vi "5492_AutonomousTurnButBetter.vi"(8 "error in (no error)":errorcluster, 10 "Yaw Goallll":dbl) -> (0 "error out (no error)":errorcluster)   [LabVIEW 2017]
uses:
  <vilib>/Rock Robotics/WPI/ThirdParty/Cross The Road Electronics/Phoenix-LabVIEW/Motor Controller/Controls/CTRE_Phoenix_MotorControl_ControlMode.ctl
  <vilib>/Rock Robotics/WPI/Utilities/WPI_GetSetVariantRefNum.vi
  5492_InitialYaw.vi
  <vilib>/Rock Robotics/WPI/RobotDrive/WPI_RobotDriveSafetyCheck.vi
  5492_DriveRamp.vi
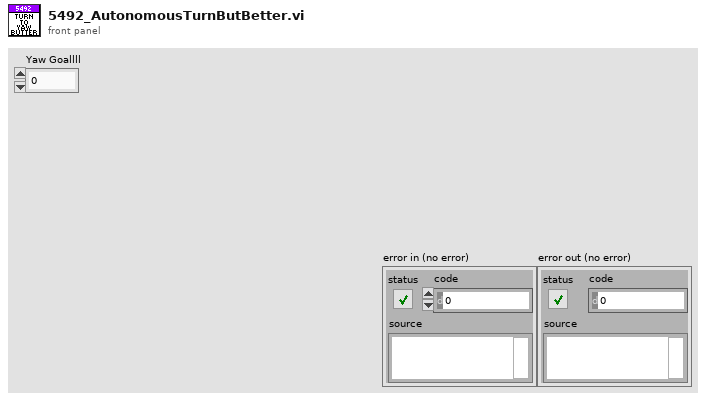
[diagram p1: front panel]
types:
  T1 = typedef "CTRE_Phoenix_MotorControl_ControlMode.ctl" = u16
  T2 = cluster{"Yaw":dbl, "Roll":dbl, "Pitch":dbl, "Heading":dbl, "Fused Heading":dbl}
  T3 = typedef "WPI_RobotDriveDevRef.ctl" = cluster{"DevStatus":errorcluster, "Motors[]":T4[], "Square Inputs":bool, "Max Output":dbl}
  T4 = typedef "WPI_MotorControlDeviceRef.ctl" = cluster{"DeviceStatus":errorcluster, "Type":T5, "PWM":cluster{"PWM Channel":T6, "DeadBand":T7}, "CAN":cluster{"Device Number":u8, "SetOutput VI Ref":variant, "GetOutput VI Ref":variant, "Enable VI Ref":variant, "Disable VI Ref":variant, "Data":variant}, "Invert":bool, "DIO PWM":cluster{"PWM \"Enable\" Channel":T6, "DIOChannel":T8, "PWM Rate":dbl}}
  T5 = typedef "WPI_MotorControlType.ctl" = enum16{"PWM", "CAN", "DIO PWM"}
  T6 = typedef "FPGA_DIOPWMChannel.ctl" = enum8{"PWM 0", "PWM 1", "PWM 2", "PWM 3", "PWM 4", "PWM 5", "PWM 6", "PWM 7", "PWM 8", "PWM 9", "PWM MXP 0", "PWM MXP 1", "PWM MXP 2", "PWM MXP 3", "PWM MXP 4", "PWM MXP 5", "PWM MXP 6", "PWM MXP 7", "PWM MXP 8", "PWM MXP 9", "Invalid"}
  T7 = typedef "WPI_PWMDeadband.ctl" = cluster{"Name":string, "maxPositivePwm":i32, "minPositivePwm":i32, "centerPwm":i32, "maxNegativePwm":i32, "minNegativePwm":i32, "angularRange":u16}
  T8 = typedef "FPGA_DIOChannel.ctl" = enum8{"DIO 0", "DIO 1", "DIO 2", "DIO 3", "DIO 4", "DIO 5", "DIO 6", "DIO 7", "DIO 8", "DIO 9", "DIO MXP 0", "DIO MXP 1", "DIO MXP 2", "DIO MXP 3", "DIO MXP 4", "DIO MXP 5", "DIO MXP 6", "DIO MXP 7", "DIO MXP 8", "DIO MXP 9", "DIO MXP 10", "DIO MXP 11", "DIO MXP 12", "DIO MXP 13", "DIO MXP 14", "DIO MXP 15", "SPI Port CS1", "SPI Port CS2", "SPI Port CS3", "SPI Port MISO", "SPI Port MOSI", "Invalid"}
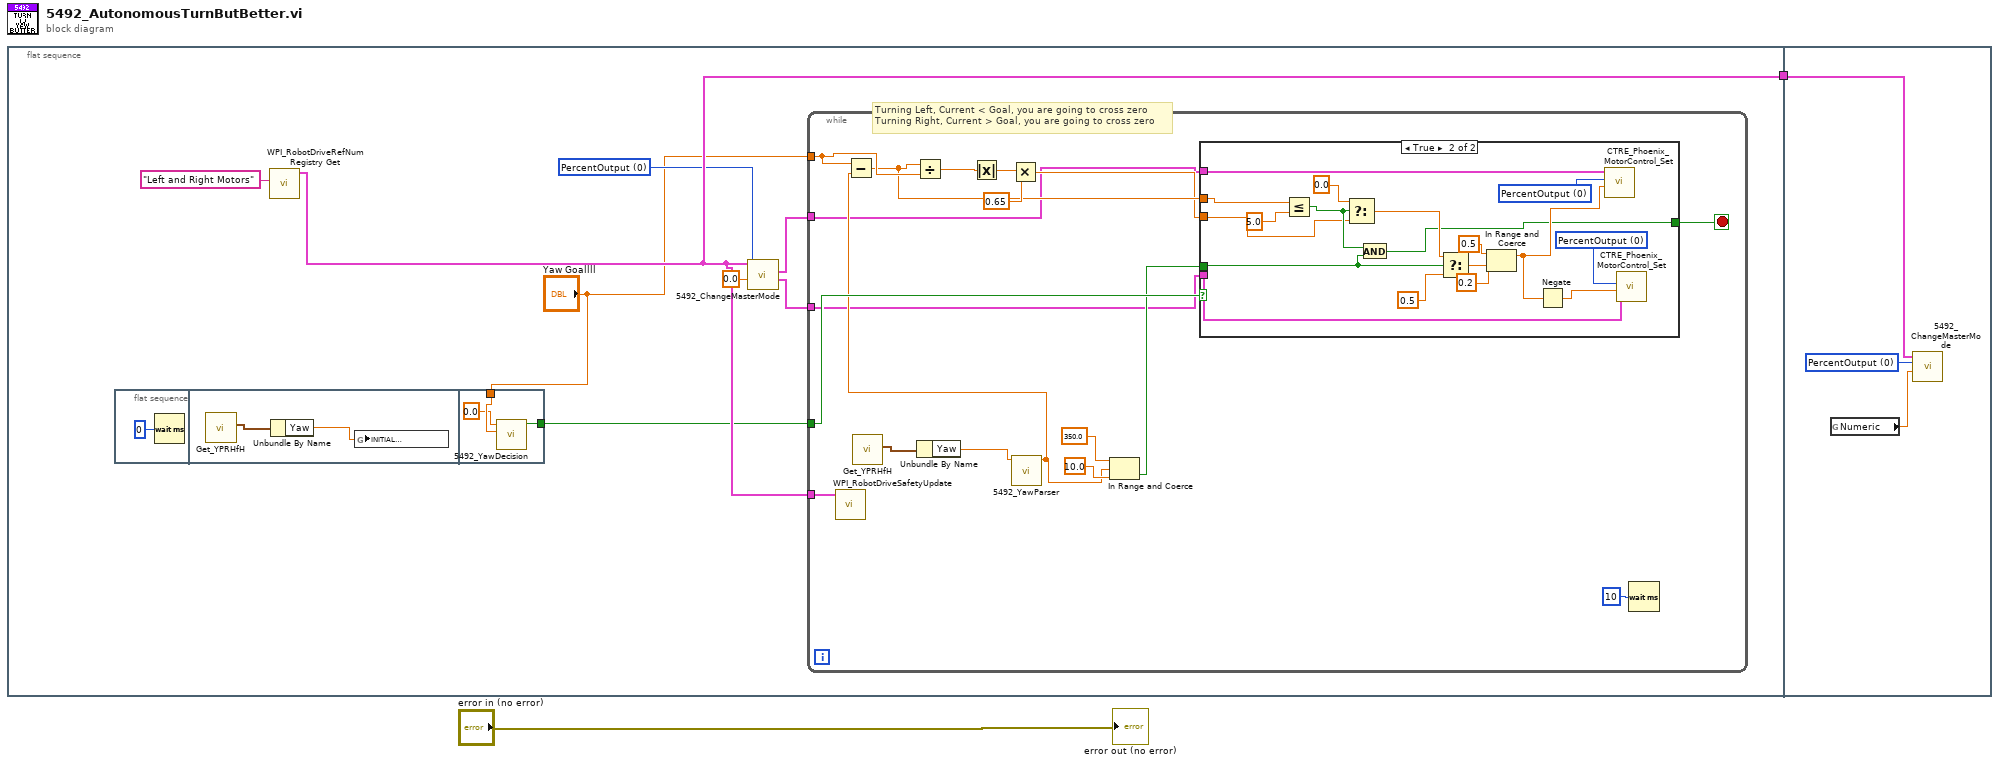
[diagram p0: block diagram]
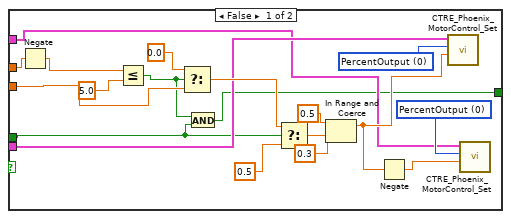
[diagram p2: hidden frame]
diagram:
  n1 = flat-sequence {
    tunnel: [w10] -> w1
    tunnel: w1 -> [w72]
    frame #0 {
      w7 = T1 0 items=["PercentOutput"=0, "Position"=1, "Velocity"=2, "Current"=3, "Follower"=5, "MotionProfile"=6, "MotionMagic"=7, "MotionMagicArc"=8, "MotionProfileArc"=10, "Disabled"=15] ("Control Mode")
      # "Turning Left, Current < Goal, you are going to cross zero\nTurning Right, Current > Goal, you are going to cross zero"
      n2 = flat-sequence {
        tunnel: "Yaw Goallll" -> [w16]
        tunnel: [w15] -> w3
        frame #0 {
          n3 = Wait (ms)(milliseconds to wait=u32 0) -> ()  [unwired: 1 out]
        }
        frame #1 {
          n4 = call <vilib>:"Get_YPRHfH.vi"() -> ("YRPHfH"=w13:T2)  [unwired: 11 in]
          n5 = Unbundle By Name(w13) -> ("Yaw"=w12:dbl)
          n6 = global write "5492_InitialYaw.vi" "INITIAL\n YAW"(w12) -> ()
        }
        frame #2 {
          n7 = call "5492_YawDecision.vi"("Yaw Goallll"=w16, "Parsed Yaw"=0.0) -> ("Right???"=w15:bool)  [unwired: 9 in]
        }
      }
      n8 = call <vilib>:"WPI_RobotDriveRefNum Registry Get.vi"("refnum name"="Left and Right Motors") -> ("RobotDriveDevRef"=w10:T3)  [unwired: 9 in, 1 out]
      n9 = call "5492_ChangeMasterMode.vi"("Ramp"=0.0, "Control Mode"=w7, "RobotDriveDevRef"=w10) -> ("CAN Talon SRX Right"=w8:T4, "CAN Talon SRX Ref Left"=w9:T4)  [unwired: 6 in, 1 out]
      n10 = while {
        tunnel: w9 -> [w19]
        tunnel: w8 -> [w18]
        tunnel: "Yaw Goallll" -> [w27]
        tunnel: w10 -> [w34]
        tunnel: w3 -> [w33]
        stop <- w20 stop-if-true
        n11 = call <vilib>:"WPI_RobotDriveSafetyUpdate.vi"("RobotDriveDevRef"=w34) -> ()  [unwired: 1 in, 10 out]
        n12 = call <vilib>:"Get_YPRHfH.vi"() -> ("YRPHfH"=w32:T2)  [unwired: 11 in]
        n13 = Unbundle By Name(w32) -> ("Yaw"=w31:dbl)
        n14 = call "5492_YawParser.vi"("Yaw"=w31) -> ("Parsed Yaw"=w28:dbl)  [unwired: 10 in]
        n15 = Subtract(x=w27, y=w28) -> (x-y=w22:dbl)
        n16 = Divide(x=w22, y=w27) -> (x/y=w26:dbl)
        n17 = Absolute Value(x=w26) -> (abs(x)=w25:dbl)
        n18 = Multiply(x=w25, y=0.65) -> (x*y=w21:dbl)
        n19 = In Range and Coerce(upper limit=350.0, x=w28, lower limit=10.0 ("y")) -> (In Range?=w23:bool)  [unwired: 1 out]
        n20 = case shown="True" w33 {
          tunnel: w23 -> [w35 w55]
          tunnel: w22 -> [w42 w70]
          tunnel: w21 -> [w40 w54]
          tunnel: [w37 w57] -> w20
          tunnel: w19 -> [w38 w63]
          tunnel: w18 -> [w39 w62]
          frame False {
            w45 = T1 0 items=["PercentOutput"=0, "Position"=1, "Velocity"=2, "Current"=3, "Follower"=5, "MotionProfile"=6, "MotionMagic"=7, "MotionMagicArc"=8, "MotionProfileArc"=10, "Disabled"=15] ("Control Mode")
            w46 = T1 0 items=["PercentOutput"=0, "Position"=1, "Velocity"=2, "Current"=3, "Follower"=5, "MotionProfile"=6, "MotionMagic"=7, "MotionMagicArc"=8, "MotionProfileArc"=10, "Disabled"=15] ("Control Mode")
            n21 = Negate(x=w42) -> (-x=w41:dbl)
            n22 = Less Or Equal?(x=w41, y=5.0) -> (x <= y?=w36:bool)
            n23 = Select(t=0.0, s=w36, f=w40) -> (s? t:f=w50:dbl)
            n24 = And(x=w36, y=w35) -> (x .and. y?=w37:bool)
            n25 = Select(t=w50, s=w35, f=0.5) -> (s? t:f=w49:dbl)
            n26 = In Range and Coerce(upper limit=0.5, x=w49, lower limit=0.3) -> (coerced(x)=w43:dbl)  [unwired: 1 out]
            n27 = Negate(x=w43) -> (-x=w44:dbl)
            n28 = call <vilib>:"CTRE_Phoenix_MotorControl_Set.vi"("Output"=w43, "Control Mode"=w45, "PhoenixMotorControlDevRef"=w39) -> ()  [unwired: 7 in, 2 out]
            n29 = call <vilib>:"CTRE_Phoenix_MotorControl_Set.vi"("Output"=w44, "Control Mode"=w46, "PhoenixMotorControlDevRef"=w38) -> ()  [unwired: 7 in, 2 out]
          }
          frame True {
            w60 = T1 0 items=["PercentOutput"=0, "Position"=1, "Velocity"=2, "Current"=3, "Follower"=5, "MotionProfile"=6, "MotionMagic"=7, "MotionMagicArc"=8, "MotionProfileArc"=10, "Disabled"=15] ("Control Mode")
            w61 = T1 0 items=["PercentOutput"=0, "Position"=1, "Velocity"=2, "Current"=3, "Follower"=5, "MotionProfile"=6, "MotionMagic"=7, "MotionMagicArc"=8, "MotionProfileArc"=10, "Disabled"=15] ("Control Mode")
            n30 = Less Or Equal?(x=w70, y=5.0) -> (x <= y?=w56:bool)
            n31 = Select(t=0.0, s=w56, f=w54) -> (s? t:f=w67:dbl)
            n32 = And(x=w56, y=w55) -> (x .and. y?=w57:bool)
            n33 = Select(t=w67, s=w55, f=0.5) -> (s? t:f=w66:dbl)
            n34 = In Range and Coerce(upper limit=0.5, x=w66, lower limit=0.2) -> (coerced(x)=w58:dbl)  [unwired: 1 out]
            n35 = Negate(x=w58) -> (-x=w59:dbl)
            n36 = call <vilib>:"CTRE_Phoenix_MotorControl_Set.vi"("Output"=w58, "Control Mode"=w60, "PhoenixMotorControlDevRef"=w63) -> ()  [unwired: 7 in, 2 out]
            n37 = call <vilib>:"CTRE_Phoenix_MotorControl_Set.vi"("Output"=w59, "Control Mode"=w61, "PhoenixMotorControlDevRef"=w62) -> ()  [unwired: 7 in, 2 out]
          }
        }
        n38 = Wait (ms)(milliseconds to wait=u32 10) -> ()  [unwired: 1 out]
      }
    }
    frame #1 {
      w73 = T1 0 items=["PercentOutput"=0, "Position"=1, "Velocity"=2, "Current"=3, "Follower"=5, "MotionProfile"=6, "MotionMagic"=7, "MotionMagicArc"=8, "MotionProfileArc"=10, "Disabled"=15] ("Control Mode")
      n39 = global read "5492_DriveRamp.vi" "Numeric"() -> (w74:dbl)
      n40 = call "5492_ChangeMasterMode.vi"("Ramp"=w74, "Control Mode"=w73, "RobotDriveDevRef"=w72) -> ()  [unwired: 6 in, 3 out]
    }
  }
  "error out (no error)" <- "error in (no error)"
